vi "Pressure.vi"(7 "Error In":errorcluster, 8 "File Path":path, 10 "Pressure":dynamicdata(graph)) -> (0 "Error Out":errorcluster, 1 "File Path Indicator":path, 2 "Interruption Time":dbl, 3 "Pressure":dbl)   [LabVIEW 2020, in "AnalysisSupport.lvlib"]
uses:
  AnalysisSupport.lvlib
  <vilib>/Waveform/WDTOps.llb/WDT Get XY Value DBL.vi
panel:
  in  "Mark Pressure":bool
  out "Enlarged":dynamicdata(graph)
  out "Pressure":dynamicdata(graph)
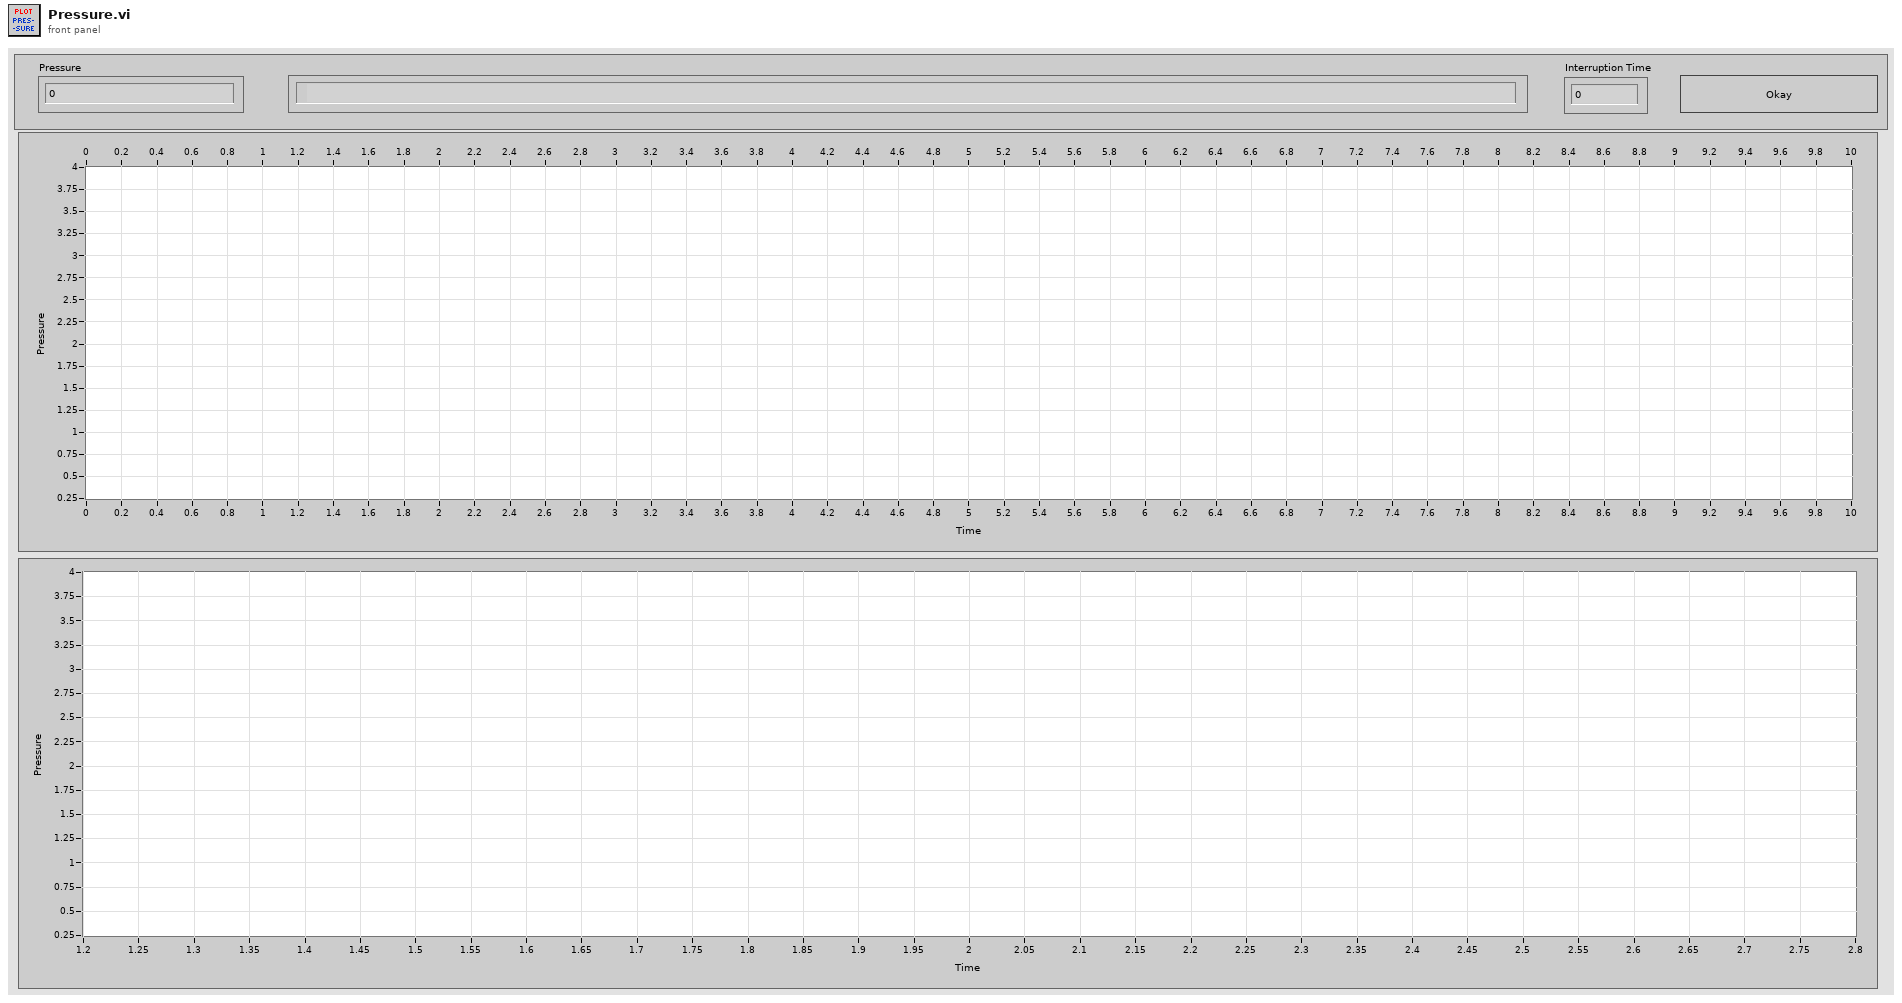
[diagram p1: front panel]
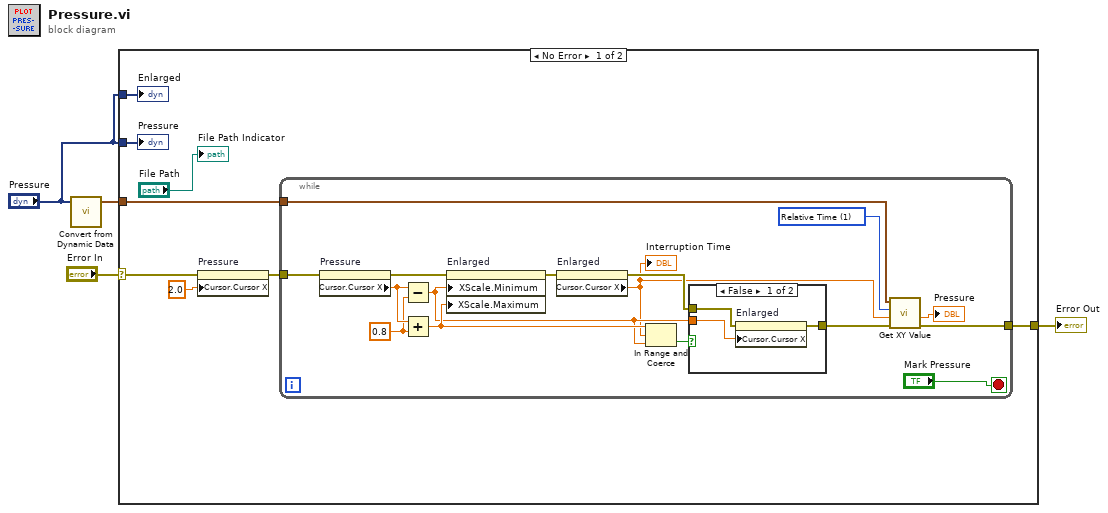
[diagram p0: block diagram]
diagram:
  n1 = call "Convert from Dynamic Data"("Dynamic Data Type"="Pressure") -> ("Waveform"=w2:waveform(dbl))  [unwired: 3 in]
  n2 = case shown="No Error" "Error In" {
    selector: "Error In" -> [w9 w33]
    tunnel: [w11 w33] -> w4
    tunnel: "Pressure" -> [w7 _]
    tunnel: "Pressure" -> [w6 _]
    tunnel: w2 -> [w5 _]
    frame No Error {
      n3 = property on="Pressure" class="WFGraph (strict)"(error in=w9, "Cursor.Cursor X"=2.0 ("Cursor.Cursor Position:Cursor X")) -> (error out=w8:errorcluster)  [unwired: 1 in, 1 out]
      n4 = while {
        tunnel: w8 -> [w22]
        tunnel: [w17] -> w11
        tunnel: w5 -> [w15]
        stop <- "Mark Pressure" stop-if-true
        w14 = u16 1 items=["Samples", "Relative Time"] ("Y position format")
        w26 = 0.8 ("y")
        n5 = property on="Pressure" class="WFGraph (strict)"(error in=w22) -> (error out=w21:errorcluster, "Cursor.Cursor X"=w27:dbl)  [unwired: 1 in, 1 out]
        n6 = Subtract(x=w27, y=w26) -> (x-y=w16:dbl)
        n7 = Add(x=w27, y=w26) -> (x+y=w25:dbl)
        n8 = property on="Enlarged" class="WFGraph (strict)"(error in=w21, "XScale.Minimum"=w16, "XScale.Maximum"=w25) -> (error out=w20:errorcluster)  [unwired: 1 in, 1 out]
        n9 = property on="Enlarged" class="WFGraph (strict)"(error in=w20) -> (error out=w19:errorcluster, "Cursor.Cursor X"=w13:dbl)  [unwired: 1 in, 1 out]
        "Interruption Time" <- w13
        n10 = In Range and Coerce(upper limit=w25, x=w13, lower limit=w16) -> (In Range?=w28:bool)  [unwired: 1 out]
        n11 = case shown="False" w28 {
          tunnel: w19 -> [w31 w32]
          tunnel: [w30 w32] -> w18
          tunnel: w16 -> [w29 _]
          frame False {
            n12 = property on="Enlarged" class="WFGraph (strict)"(error in=w31, "Cursor.Cursor X"=w29) -> (error out=w30:errorcluster)  [unwired: 1 in, 1 out]
          }
          frame True {
          }
        }
        n13 = call-poly <vilib>:"Get XY Value.vi"("error in (no error)"=w18, "Y position"=w13, "Y position format"=w14, "waveform in"=w15) -> ("error out"=w17:errorcluster, "Y value"=→"Pressure":dbl)  [unwired: 3 in, 3 out]
      }
      "File Path Indicator" <- "File Path"
      "Enlarged" <- w6
      "Pressure" <- w7
    }
    frame Error {
    }
  }
  "Error Out" <- w4
